vi "Launch_Actor.vi"(8 "error in":errorcluster, 11 "vi reference":refnum<vi>) -> (0 "error out":errorcluster)   [LabVIEW 2010]
doc: "This VI implements the routine for launching actors using a reference. Once the actor is launched it will register its communication queue using a global variable for further communcaition with the other actors within the paralllel environment.\n\ncreated by Davis Montenegro\nEPRI\n04-23-2017"
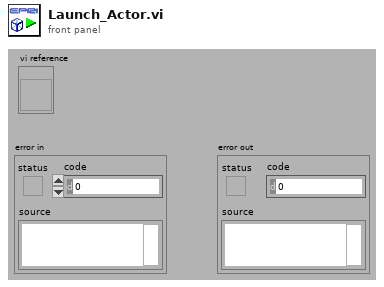
[diagram p1: front panel]
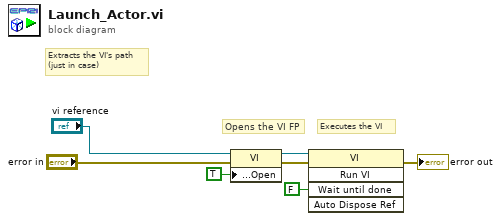
[diagram p0: block diagram]
diagram:
  # "Executes the VI"
  # "Opens the VI FP"
  # "Extracts the VI's path\n(just in case)"
  n1 = property class="VI"(reference="vi reference", error in="error in", "Front Panel.Open"=TRUE ("Front Panel Window:Open")) -> (reference out=w4:refnum<vi>, error out=w5:errorcluster)
  n2 = invoke class="VI" method="Run VI"(reference=w4, error in=w5, "Wait until done"=FALSE ("Wait Until Done")) -> (error out=→"error out":errorcluster)  [unwired: 2 in, 4 out]
